vi "Move to Level.vi"(8 "error in (no error)":errorcluster, 10 "Element":string, 11 "json class in":refnum<class "json class.lvclass">) -> (0 "error out":errorcluster, 2 "New json class":refnum<class "json class.lvclass">, 3 "json class out":refnum<class "json class.lvclass">)   [LabVIEW 2025, in "Config Library.lvlib" / "json class.lvclass"]
uses:
  json class.lvclass
  <vilib>/addons/JSON API/JSON Value/JSON Value.lvclass
  json class.lvclass/json class.ctl
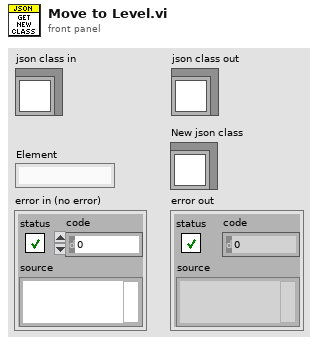
[diagram p1: front panel]
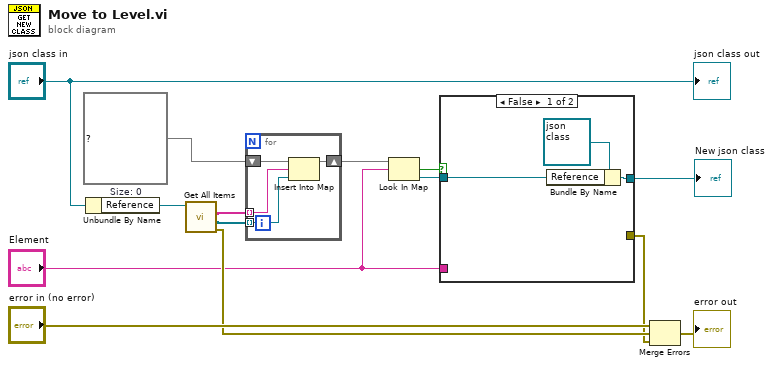
[diagram p0: block diagram]
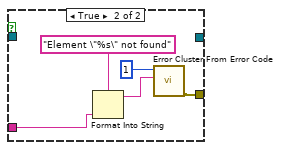
[diagram p2: hidden frame]
diagram:
  w11 = map{string, refnum<class "JSON Value.lvclass">} {}  # Size: 0
  n1 = Unbundle By Name("json class in") -> ("Reference"=w12:refnum<class "JSON Value.lvclass">)
  n2 = call-dynamic "Get All Items.vi"("JSON Value In"=w12) -> ("error out"=w6:errorcluster, "Values"=w9:refnum<class "JSON Value.lvclass">[], "Item Names"=w10:string[])  [unwired: 7 in, 1 out]
  n3 = for {
    tunnel: w10 -> [w16] mode=indexing
    tunnel: w9 -> [w15] mode=indexing
    shift-right: [w17] -> w13
    shift-left: w11 -> [w18]
    n4 = Insert Into Map(map in=w18, key=w16, value=w15) -> (map out=w17:map{string, refnum<class "JSON Value.lvclass">})  [unwired: 2 out]
  }
  n5 = Look In Map(map=w13, key="Element") -> (key not found?=w4:bool, value=w14:refnum<class "JSON Value.lvclass">)  [unwired: 1 in]
  n6 = case shown="False" w4 {
    tunnel: w14 -> [w21 _]
    tunnel: [w20 _] -> w2
    tunnel: [_ w26] -> w5
    tunnel: "Element" -> [_ w22]
    frame False {
      n7 = Bundle By Name(cluster=refnum<class "json class.lvclass"> refnum ("Config Library.lvlib:json class.lvclass"), "Reference"=w21) -> (w20:refnum<class "json class.lvclass">)
    }
    frame True {
      n8 = Format Into String(format string="Element \"%s\" not found" ("error message (\"\")"), w22) -> (resulting string=w23:string)  [unwired: 2 in, 1 out]
      n9 = call <vilib>:"Error Cluster From Error Code.vi"("error message (\"\")"=w23, "error code (0)"=1) -> ("error out"=w26:errorcluster)  [unwired: 7 in]
    }
  }
  "New json class" <- w2
  n10 = Merge Errors("error in (no error)", w6, w5) -> (→"error out":errorcluster)
  "json class out" <- "json class in"
